vi "Configure Messages.vi"(8 "error in (no error)":errorcluster, 10 "Messages":string[](array[string]), 11 "Debugger In":refnum<class "Debugger.lvclass">) -> (0 "error out":errorcluster, 3 "Debugger Out":refnum<class "Debugger.lvclass">)   [LabVIEW 2020, in "Debugger.lvclass"]
uses:
  Debugger.lvclass
  C:/Users/anton/Documents/GitHub/triarc-debugger/source/Process/Debug Process.lvclass
  Process/Debug Process.lvclass/Debug Process.ctl
  Debugger.lvclass/Debugger.ctl
  <vilib>/Utility/error.llb/Clear Errors.vi
  Filter by Message/Filter by Message.lvclass
  C:/Users/anton/Documents/GitHub/triarc-debugger/source/Filter/Filter.lvclass
  <vilib>/Utility/error.llb/Error Cluster From Error Code.vi
  Process/Debug Process.lvclass
  Debug Log/Debug Log.lvclass
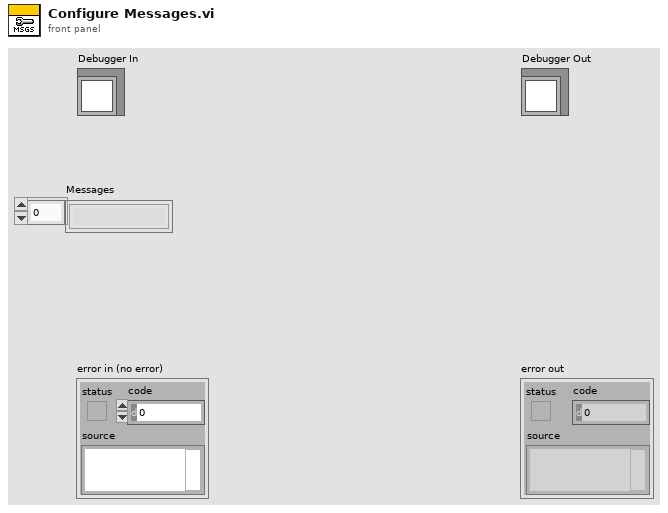
[diagram p1: front panel]
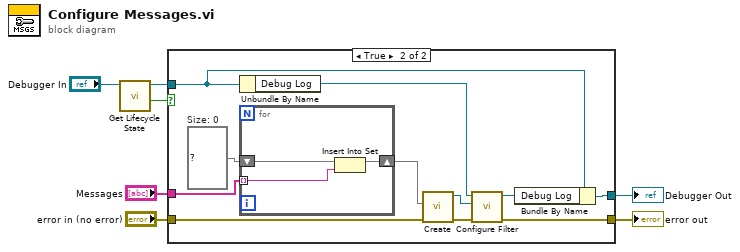
[diagram p0: block diagram]
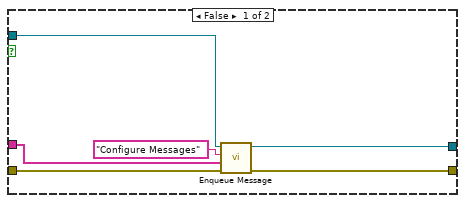
[diagram p2: hidden frame]
diagram:
  n1 = call "Get Lifecycle State.vi"("Process In"="Debugger In") -> ("In Process Loop?"=w1:bool, "Process Out"=w2:refnum<class "Debugger.lvclass">)  [unwired: 7 in, 2 out]
  n2 = case shown="True" w1 {
    tunnel: "error in (no error)" -> [w13 w21]
    tunnel: [w12 w20] -> w6
    tunnel: [w11 w23] -> w4
    tunnel: "Messages" -> [w9 w22]
    tunnel: w2 -> [w8 w24]
    frame False {
      n3 = call "Enqueue Message.vi"("error in (no error)"=w13, "Message Data"=w9, "Message"="Configure Messages", "Process In"=w8) -> ("error out"=w12:errorcluster, "Process Out"=w11:refnum<class "Debugger.lvclass">)  [unwired: 6 in]
    }
    frame True {
      w18 = set{string} {}  # Size: 0
      n4 = Unbundle By Name(w24) -> ("Debug Log"=w17:refnum<class "Debug Log.lvclass">)
      n5 = for {
        shift-right: [w26] -> w19
        shift-left: w18 -> [w27]
        tunnel: w22 -> [w25] mode=indexing
        n6 = Insert Into Set(10:w25, 11:w27) -> (3:w26:set{string})  [unwired: 1 out]
      }
      n7 = call "Create.vi"("error in (no error)"=w21, "Messages"=w19) -> ("error out"=w15:errorcluster, "Filter by Process out"=w16:refnum<class "Filter by Message.lvclass">)  [unwired: 8 in]
      n8 = call "Configure Filter.vi"("error in (no error)"=w15, "Filter"=w16, "Debug Log In"=w17) -> ("error out"=w20:errorcluster, "Debug Log Out"=w14:refnum<class "Debug Log.lvclass">)  [unwired: 7 in]
      n9 = Bundle By Name(cluster=w24, "Debug Log"=w14) -> (w23:refnum<class "Debugger.lvclass">)
    }
  }
  "error out" <- w6
  "Debugger Out" <- w4
